vi "GT Get Trigger Status.vi"(7 "count":i16, 8 "error in (no error)":errorcluster caption="错误输入（无错误）", 9 "pTriggerStatus":T1, 10 "i":i16, 11 "cardNum":i16) -> (0 "error out":errorcluster caption="错误输出", 1 "pTriggerStatus out":T1, 3 "function return":i16)   [LabVIEW 2020, in "gts.lvlib"]
doc: "GT_API GT_GetTriggerStatus(short cardNum,short i,TTriggerStatus *pTriggerStatus,short count=1);"
uses:
  gts.lvlib
  dll/32bit/multi_card/gts.dll
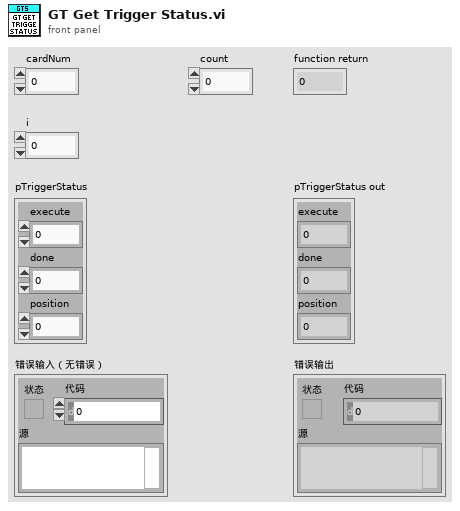
[diagram p1: front panel]
types:
  T1 = cluster{"execute":i16, "done":i16, "position":i32}
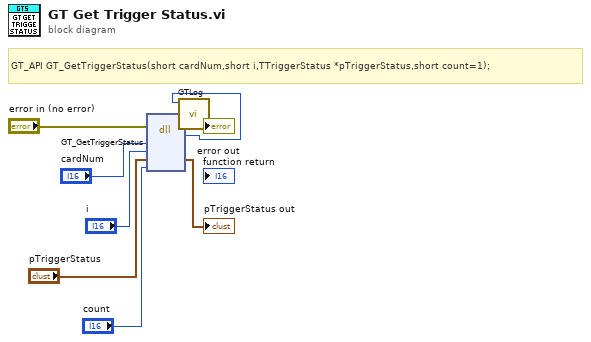
[diagram p0: block diagram]
diagram:
  # "GT_API GT_GetTriggerStatus(short cardNum,short i,TTriggerStatus *pTriggerStatus,short count=1);"
  n1 = dll-call lib="C:/1228/dll/32bit/multi_card/gts.dll" fn="GT_GetTriggerStatus"(error in="error in (no error)", "cardNum"="cardNum", "i"="i", "pTriggerStatus"="pTriggerStatus", "count"="count") -> (error out=w3:errorcluster, w1:i16, "pTriggerStatus"=→"pTriggerStatus out":T1)  [unwired: 5 in, 1 out]
  n2 = call "GTLog.vi"("error in (no error)"=w3, "Numeric"=w1) -> ("error out"=→"error out":errorcluster)  [unwired: 9 in]
